vi "Log_Partitioned.vi"(10 "Array":sgl[](array[numeric]), 11 "Byte Stream File in":refnum<file>) -> (3 "Byte Stream File out":refnum<file>)   [LabVIEW 2020]
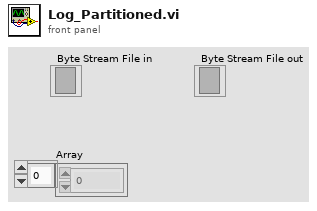
[diagram p1: front panel]
types:
  T1 = cluster{"Array[0]":sgl, "Array[1]":sgl, "Array[2]":sgl, "Array[3]":sgl, "Array[4]":sgl, "Array[5]":sgl, "Array[6]":sgl, "Array[7]":sgl, "Array[8]":sgl}
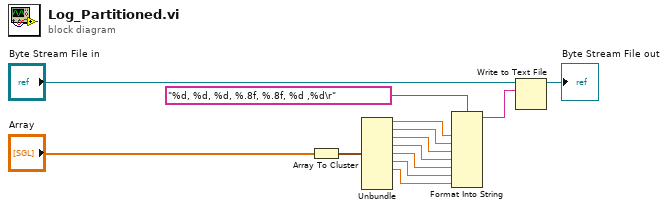
[diagram p0: block diagram]
diagram:
  n1 = Array To Cluster(array="Array") -> (cluster=w4:T1)
  n2 = Unbundle(w4) -> ("Array[0]"=w5:sgl, "Array[1]"=w6:sgl, "Array[2]"=w7:sgl, "Array[3]"=w8:sgl, "Array[4]"=w9:sgl, "Array[5]"=w10:sgl, "Array[6]"=w11:sgl)  [unwired: 2 out]
  n3 = Format Into String(format string="%d, %d, %d, %.8f, %.8f, %d ,%d\r", w5, w6, w7, w8, w9, w10, w11) -> (resulting string=w13:string)  [unwired: 2 in, 1 out]
  n4 = Write to Text File(file (use dialog)="Byte Stream File in", text=w13) -> (refnum out=→"Byte Stream File out":refnum<file>)  [unwired: 2 in, 2 out]
